vi "Stop Core.vi"(10 "final error code":i32, 11 "Actor1_GUI in":refnum<class "Actor1_GUI_N_4.0.0.lvclass">) -> (3 "Actor1_GUI out":refnum<class "Actor1_GUI_N_4.0.0.lvclass">)   [LabVIEW 2020, in "Actor1_GUI_N_4.0.0.lvlib" / "Actor1_GUI_N_4.0.0.lvclass"]
doc: "(<B>Filename</B>: Actor Framework.lvlib:Actor.lvclass:Stop Core.vi)\n\nDefines what the actor does before it stops. Use the <B>final error code</B> input to determine whether the actor shut down in response to an error.\n\nBy default, this method does nothing. A descendant class may override it to define behavior, such as shutting down any processes the actor initiated in its override of the Actor Core method."
uses:
  <resource>/Framework/Providers/Open_GDS/ClassProviders/ActorFramework/4.0.0/Actor1_GUI_N_4.0.0/Actor1_GUI_N_4.0.0_class/Actor1_GUI_N_4.0.0.lvclass
  <resource>/Framework/Providers/Open_GDS/ClassProviders/ActorFramework/4.0.0/Actor1_GUI_N_4.0.0/Actor1_GUI_N_4.0.0_class/Actor1_GUI_N_4.0.0.lvclass/Actor1_GUI_N_4.0.0.ctl
  <vilib>/ActorFramework/Actor/Actor.lvclass
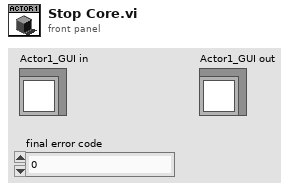
[diagram p1: front panel]
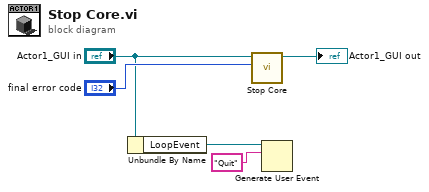
[diagram p0: block diagram]
diagram:
  n1 = Unbundle By Name("Actor1_GUI in") -> ("LoopEvent"=w2:refnum<user-event>)
  n2 = call-parent "Stop Core.vi"("final error code"="final error code", "Actor in"="Actor1_GUI in") -> ("Actor out"=→"Actor1_GUI out":refnum<class "Actor1_GUI_N_4.0.0.lvclass">)  [unwired: 9 in]
  n3 = Generate User Event(user event=w2, event data cluster="Quit" ("event data")) -> ()  [unwired: 2 in, 2 out]
